vi "New Network Session Handler.vi"(7 "Retry Timeout":i32, 8 "error in (no error)":errorcluster, 9 "Log Instance Reference":refnum<class "LoggerReference.lvclass">, 10 "MessageProtocol":refnum<class "IMessagingProtocol.lvclass">, 11 "Connection Factory Type":refnum<class "IConnectionFactory.lvclass">) -> (0 "error out":errorcluster, 3 "Session Queue":refnum<queue>)   [LabVIEW 2019, in "Network Sink.lvlib" / "SessionHandler.lvclass"]
uses:
  <vilib>/gpm_packages/@cs/event-logger/Source/Network Sink/SessionHandler/SessionHandler.lvclass
  <vilib>/gpm_packages/@cs/Network-Sink/Source/Network Interface/IMessagingProtocol/IMessagingProtocol.lvclass
  <vilib>/gpm_packages/@cs/Network-Sink/Source/Network Interface/IConnectionFactory/IConnectionFactory.lvclass
  <vilib>/gpm_packages/@cs/event-logger/Source/Composed Log/LoggerReference/LoggerReference.lvclass
  <vilib>/gpm_packages/@cs/event-logger/Source/Network Sink/SessionHandler/SessionHandler.lvclass/SessionHandler.ctl
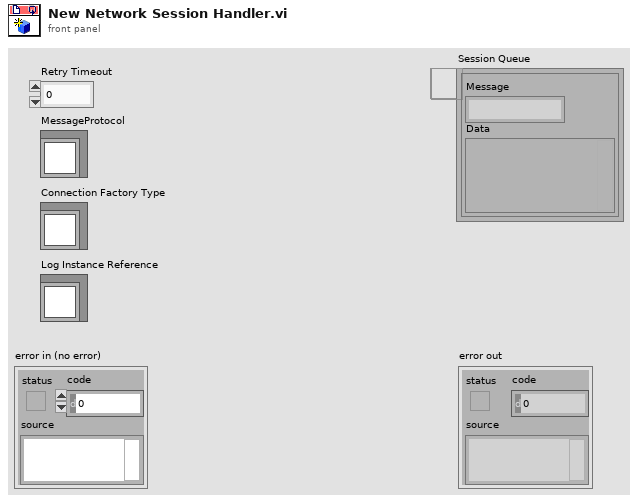
[diagram p1: front panel]
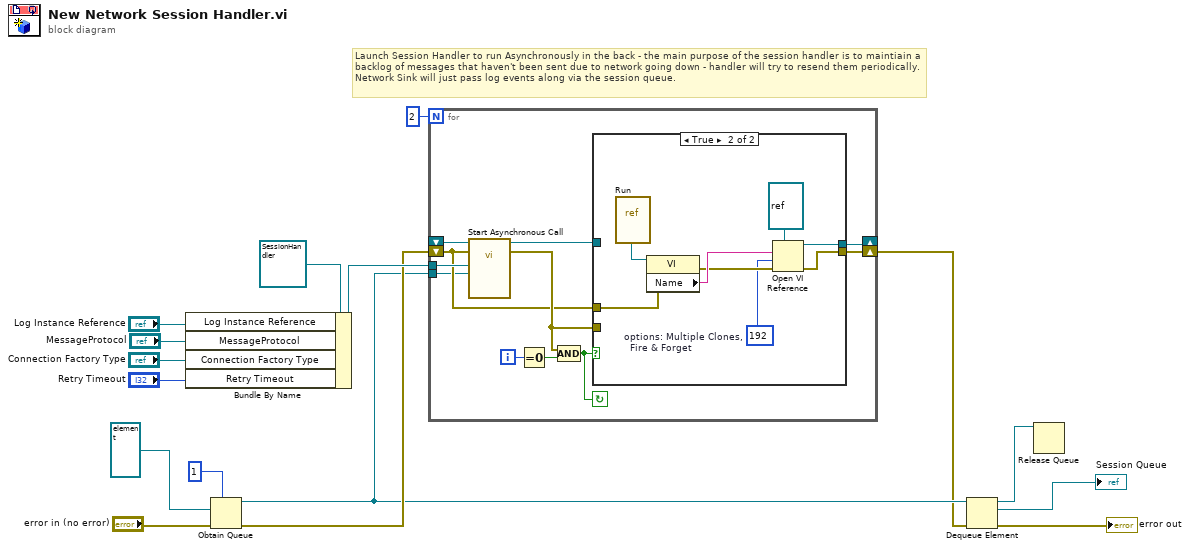
[diagram p0: block diagram]
diagram:
  # "Launch Session Handler to run Asynchronously in the back - the main purpose of the session handler is to maintiain a backlog of messages that haven't been sent due to network going down - handler will try to resend them periodically. Network Sink will just pass log events along via the session queue."
  n1 = Bundle By Name(cluster=refnum<class "SessionHandler.lvclass"> refnum ("SessionHandler in"), "Log Instance Reference"="Log Instance Reference", "MessageProtocol"="MessageProtocol", "Connection Factory Type"="Connection Factory Type", "Retry Timeout"="Retry Timeout") -> (w15:refnum<class "SessionHandler.lvclass">)
  n2 = Obtain Queue(max queue size (-1, unlimited)=1, element data type=refnum<queue> refnum ("Self Queue"), error in (no error)="error in (no error)") -> (queue out=w9:refnum<queue>, error out=w10:errorcluster)  [unwired: 2 in, 1 out]
  n3 = for {
    N: 2 -> [_]
    tunnel: w15 -> [w20]
    shift-right: [w26] -> _
    shift-left: _ -> [w27]
    shift-right: [w21] -> w8
    shift-left: w10 -> [w19]
    tunnel: w9 -> [w18]
    i -> [w23]
    stop <- w17 continue-if-true
    n4 = call-by-ref "Start Asynchronous Call"(reference=w27, error in=w19, "Return Queue"=w18, "SessionHandler in"=w20) -> (reference out=w25:refnum<vi>, error out=w22:errorcluster)  [unwired: 10 in]
    n5 = Equal To 0?(x=w23) -> (x = 0?=w24:bool)
    n6 = Compound Arithmetic op=AND(w22, w24) -> (w17:bool)
    n7 = case shown="True" w17 {
      tunnel: [w29 w34] -> w26
      tunnel: w25 -> [w29 _]
      tunnel: w22 -> [w28 _]
      tunnel: [w28 w32] -> w21
      tunnel: w19 -> [_ w31]
      frame False {
      }
      frame True {
        w30 = 192  # options: Multiple Clones,   Fire & Forget
        n8 = vi-ref <vilib>:"Run.vi"() -> (w37:refnum<vi>)
        n9 = property class="VI"(reference=w37, error in=w31) -> (error out=w33:errorcluster, "Name"=w36:string)  [unwired: 1 out]
        n10 = Open VI Reference(type specifier VI Refnum (for type only)=refnum<vi> refnum, vi path=w36, options=w30, error in (no error)=w33) -> (vi reference=w34:refnum<vi>, error out=w32:errorcluster)  [unwired: 2 in]
      }
    }
  }
  n11 = Dequeue Element(queue=w9, error in (no error)=w8) -> (queue out=w7:refnum<queue>, element=→"Session Queue":refnum<queue>, error out=→"error out":errorcluster)  [unwired: 1 in, 1 out]
  n12 = Release Queue(queue=w7) -> ()  [unwired: 2 in, 3 out]
